vi "Configure Load Trigger.vi"(0 "VISA resource name":refnum<visa-resource-name>, 1 "Templates (0: DurationLoop)":i32(ring) items=["DurationLoop", "LogicTrigger", "LoopUntilEvent", "SimpleLoop"], 2 "Duration (1)":dbl=1.0, 3 "Dig Line Input (1)":i32=1, 4 "Dig Line Output (2)":i32=2, 5 "error in (no error)":errorcluster, 6 "Clear (Never)":i32(ring)=1 items=["Enter", "Never"], 7 "Delay (0)":dbl, 8 "Buffer Name (0: defbuffer1)":i32(ring) items=["defbuffer1", "defbuffer2"], 9 "Count (1)":i32=1, 10 "Event Constant (27: Blender 1)":u16(ring)=27 items=["Display", "Notify 1", "Notify 2", "Notify 3", "Notify 4", "Notify 5", "Notify 6", "Notify 7", "Notify 8", "Command", "Dig 1", "Dig 2", "Dig 3", "Dig 4", "Dig 5", "Dig 6", "LAN1", "LAN2", "LAN3", "LAN4", "LAN5", "LAN6", "LAN7", "LAN8", "Tsplink1", "Tsplink2", "Tsplink3", "Blender1", "Blender2", "Timer1", "Timer2", "Timer3", "Timer4", "Atrigger", "External"], 11 "Position (0)":i32) -> (14 "VISA resource name out":refnum<visa-resource-name>, 19 "error out":errorcluster)   [LabVIEW 2023, in "Keithley DMM6500 DAQ6500 Series.lvlib"]
doc: "Load the trigger with the arguments"
uses:
  <instrlib>/Keithley DMM6500 DAQ6500 Series/Keithley DMM6500 DAQ6500 Series.lvlib
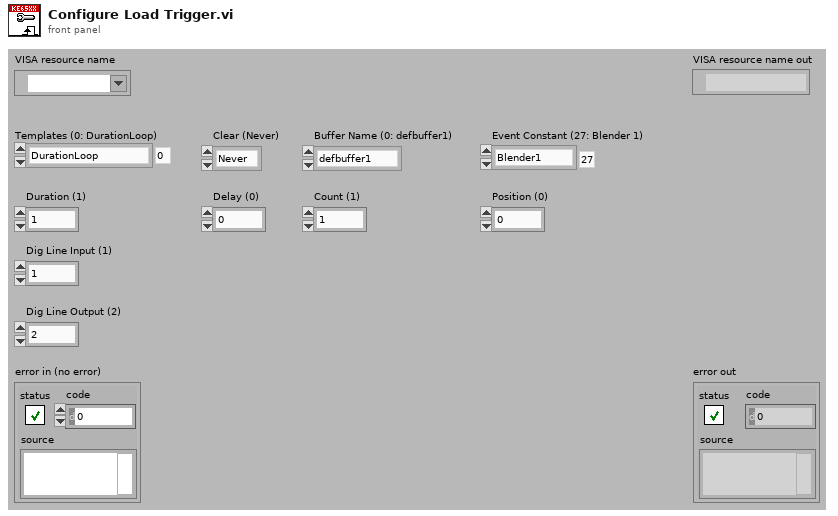
[diagram p1: front panel]
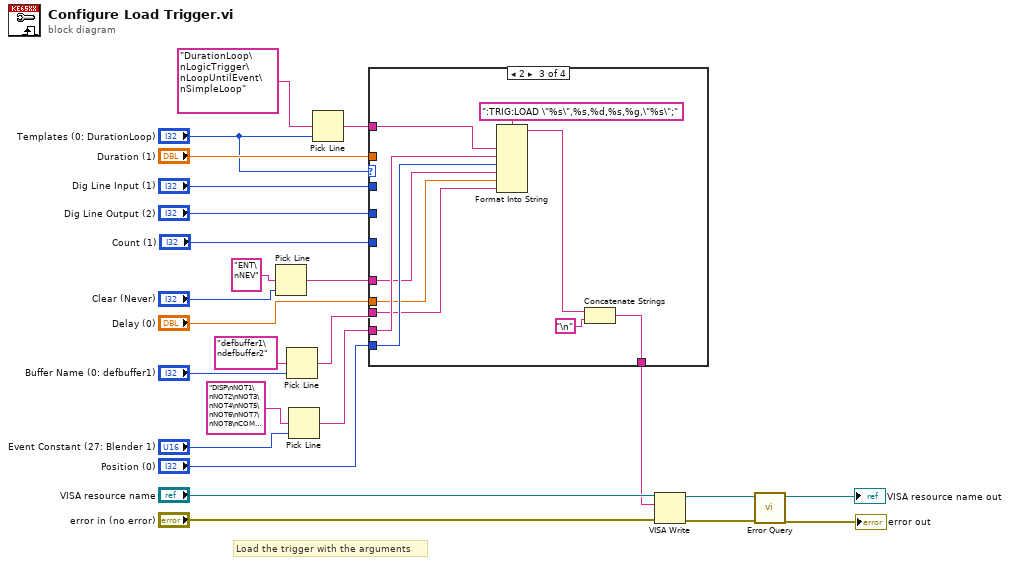
[diagram p0: block diagram]
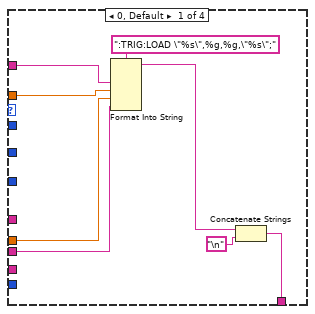
[diagram p2: hidden frame]
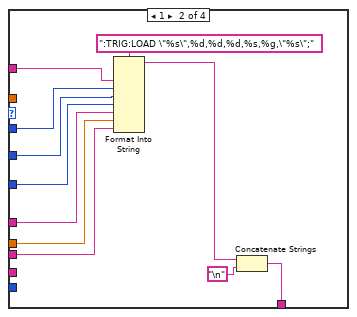
[diagram p3: hidden frame]
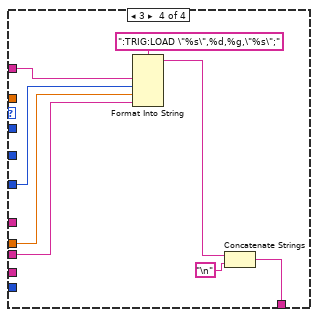
[diagram p4: hidden frame]
diagram:
  # "Load the trigger with the arguments"
  n1 = Pick Line(multi-line string="ENT\nNEV", line index="Clear (Never)") -> (output string=w6:string)  [unwired: 1 in]
  n2 = Pick Line(multi-line string="defbuffer1\ndefbuffer2", line index="Buffer Name (0: defbuffer1)") -> (output string=w9:string)  [unwired: 1 in]
  n3 = Pick Line(multi-line string="DISP\nNOT1\nNOT2\nNOT3\nNOT4\nNOT5\nNOT6\nNOT7\nNOT8\nCOMM\nDIG1\nDIG2\nDIG3\nDIG4\nDIG5\nDIG6\nLAN1\nLAN2\nLAN3\nLAN4\nLAN5\nLAN6\nLAN7\nLAN8\nTSP1\nTSP2\nTSP3\nBLEN1\nBLEN2\nTIM1\nTIM2\nTIM3\nTIM4\nATR\nEXT", line index="Event Constant (27: Blender 1)") -> (output string=w2:string)  [unwired: 1 in]
  n4 = Pick Line(multi-line string="DurationLoop\nLogicTrigger\nLoopUntilEvent\nSimpleLoop", line index="Templates (0: DurationLoop)") -> (output string=w19:string)  [unwired: 1 in]
  n5 = case shown="2" "Templates (0: DurationLoop)" {
    tunnel: w19 -> [w32 w43 w53 w61]
    tunnel: [w31 w42 w52 w60] -> w17
    tunnel: "Duration (1)" -> [w28 _ _ _]
    tunnel: "Delay (0)" -> [w27 w36 w46 w56]
    tunnel: w9 -> [w26 w35 w45 w55]
    tunnel: "Dig Line Input (1)" -> [_ w39 _ _]
    tunnel: "Count (1)" -> [_ w38 _ w57]
    tunnel: w6 -> [_ w37 w47 _]
    tunnel: w2 -> [_ _ w49 _]
    tunnel: "Position (0)" -> [_ _ w48 _]
    tunnel: "Dig Line Output (2)" -> [_ w34 _ _]
    frame 0, Default {
      n6 = Format Into String(format string=":TRIG:LOAD \"%s\",%g,%g,\"%s\";", w32, w28, w27, w26) -> (resulting string=w30:string)  [unwired: 2 in, 1 out]
      n7 = Concatenate Strings(w30, "\n") -> (w31:string)
    }
    frame 1 {
      n8 = Format Into String(format string=":TRIG:LOAD \"%s\",%d,%d,%d,%s,%g,\"%s\";", w43, w39, w34, w38, w37, w36, w35) -> (resulting string=w41:string)  [unwired: 2 in, 1 out]
      n9 = Concatenate Strings(w41, "\n") -> (w42:string)
    }
    frame 2 {
      n10 = Format Into String(format string=":TRIG:LOAD \"%s\",%s,%d,%s,%g,\"%s\";", w53, w49, w48, w47, w46, w45) -> (resulting string=w51:string)  [unwired: 2 in, 1 out]
      n11 = Concatenate Strings(w51, "\n") -> (w52:string)
    }
    frame 3 {
      n12 = Format Into String(format string=":TRIG:LOAD \"%s\",%d,%g,\"%s\";", w61, w57, w56, w55) -> (resulting string=w59:string)  [unwired: 2 in, 1 out]
      n13 = Concatenate Strings(w59, "\n") -> (w60:string)
    }
  }
  n14 = VISA Write(VISA resource name="VISA resource name", write buffer=w17, error in (no error)="error in (no error)") -> (VISA resource name out=w23:refnum<visa-resource-name>, error out=w22:errorcluster)  [unwired: 1 out]
  n15 = call <instrlib>:"Error Query.vi"("error in (no error)"=w22, "VISA resource name"=w23) -> ("error out"=→"error out":errorcluster, "VISA resource name out"=→"VISA resource name out":refnum<visa-resource-name>)  [unwired: 6 in, 2 out]
